vi "AOD Control (host).vi"() -> ()   [LabVIEW 2012]
uses:
  <vilib>/rvi/interface/nirviOpenFPGA/nirviOpenFPGA.xnode
  <vilib>/rvi/interface/nirviReadWriteControl/nirviReadWriteControl.xnode
  <vilib>/rvi/interface/nirviMethod/nirviMethod.xnode
  <vilib>/LabVIEW Targets/FPGA/RIO/nirio_PxiTriggers.ctl
  <vilib>/rvi/interface/nirviCloseFPGA/nirviCloseFPGA.xnode
  <resource>/objmgr/daqmx.rc
  <vilib>/Utility/error.llb/DialogType.ctl
  <vilib>/DAQmx/write.llb/DAQmx Write (Digital Bool 1Line 1Point).vi
  <instrlib>/niHWS/nihws.llb/niHWS Write Analog I32.vi
  <instrlib>/niHWS/nihws.llb/niHWS Open File Permissions ID.ctl
  <vilib>/DAQmx/create/channels.llb/DAQmx Create Channel (DO-Digital Output).vi
  <vilib>/DAQmx/read.llb/DAQmx Read (Raw 1D I32).vi
  <instrlib>/niHWS/nihws.llb/niHWS Write Analog I16.vi
  <vilib>/DAQmx/write.llb/DAQmx Write (Analog DBL 1Chan 1Samp).vi
  FPGA Bitfiles/AOD Control.lvproj_PXI-7954R_AOD Control (FPGA)~D2.lvbitx
  AOD Control (FPGA).vi
  AODRef.ctl
  <vilib>/Analysis/NI_AALBase.lvlib
  <vilib>/Analysis/1siggen.llb/Ramp Pattern by Samples.vi
  <vilib>/rvi/errors/niLvFpgaMergeErrorWithErrorCode.vi
  <vilib>/FPGA/interface/niFpgaViExecutionMode.ctl
  <vilib>/userdefined/High Color/nirio_resource_hc.ctl
panel:
  in  "Max":u32=700000
  in  "GridPoints":dbl=5.0
  in  "Power":dbl(slide) min=0.0 max=5.0 step=0.1 scale=0.0..5.0
  out "OutOfRange":bool
  out "Processing":bool
  out "Acquire":bool
  out "FPGA State":T1(ring)
  out "Host State":T2(ring)
  out "Scanning Your Mom":dbl(slide) scale=0.0..1.0
  in  "Tab Control":T3(tab)=enum."Miscellaneous"
  in  "Display Data":bool=TRUE
  in  "ClearPoints":bool
  in  "Scan Settings":T4={"XStart"=-200000000, "XEnd"=200000000, "XNum"=500, "YStart"=-200000000, "YEnd"=200000000, "YNum"=500, "ZStart"=0, "ZEnd"=0, "ZNum"=1}
  in  "Points":i32[][](array[numeric])
  in  "Stop":bool
  in  "Scan":bool
  in  "Volume Scan":bool
  in  "Abort":bool
  in  "Reset":bool
  out "Writing":bool
  in  "SaveStream":bool
  in  "SaveImage":bool
  in  "Path":path
  in  "Scans":i32=5
  in  "ImCh1":bool=TRUE
  in  "Ephys":bool
  in  "Photodiode":bool
  in  "ImCh2":bool
  in  "Throwaway (us)":i32=10
  out "PointArray":cluster{"X":i32, "Y":i32, "Z":i32}[](array[cluster])
  out "StreamInfo":T5
  in  "Downsample":i32=40
  in  "DDS SysClk":i32=100000000
  in  "FPGA Clk":i32=40000000
  in  "ImReadSize":i32=10000
  in  "AcqDivider":i32=20
  out "Acq Freq":dbl format="%#_8g"
  out "Loop Count":i32
  out "PointTime":u32
  out "PMT FIFO Space":u32
  out "ImCh Backlog":u32
  out "FPGA PMT Remaining":u32
  out "PMT Backlog":u32
  out "Command":i16
  in  "P high":u32=10
  in  "P":bool
  out "PMT Read":i32
  out "FPGA Loop Count":i32
  out "Point":cluster{"X":i32, "Y":i32, "Z":i32}
  out "TotalSamples":u32
  out "Written":cluster{"Address":u8, "Value":u32}[](array[cluster]) {"Address" format="%x"; "Value" format="%x"}
  out "PMT Array":i32[](array[numeric])
  out "ImCh Read":i32
  out "Mode":enum16{"Points", "Volume", "Idle"}(ring)
  out "FPGA VI Execution Mode":T6
  out "StackSize":cluster{"nX":u32, "nY":u32, "nZ":u32}
  out "raw out":refnum<queue>
  out "voxel queue":refnum<queue>
  out "NumChans":u32
  out "XPos":i32[](array[numeric])
  out "TRIG0":bool
  out "ExtAcqTrig":bool
  out "TriggerAcq":bool=TRUE
  out "Armed":bool
  out "Bad PMTData":bool
  out "SerialError":bool
  out "Sequencing error":bool
  out "YPos":i32[](array[numeric])
  out "ZPos":i32[](array[numeric])
  out "Point Freq":dbl
  out "SampleCount":u32
  out "AcqDivCount":u32
  out "# pending remove":i32
  out "Processed":i32
  in  "BlankTime (us)":i16=10
  out "BlankSamples":u32
  out "Throwaway Samples":dbl
  out "RepNum":i32
  out "NumReps":i32
  out "NumPoints":i32
  out "PointNum":u32
  out "LaserPowerTask":refnum<k21>
  in  "Execute":bool
  in  "Debug Mode":T7(ring)
  in  "Space":i32
  in  "decimating factor":i32=10
  in  "BaselineRate":dbl=0.01 min=0.0 max=1.0
  in  "RIO Device":T8="RIO0"
  out "ImData":i32[][](array[numeric])
  out "ImCh1 2":T9(plugin-control)
  out "ImCh2 2":T9(plugin-control)
  in  "Section":i32(c297)
  out "Waveform Chart":waveform(dbl)[](graph)
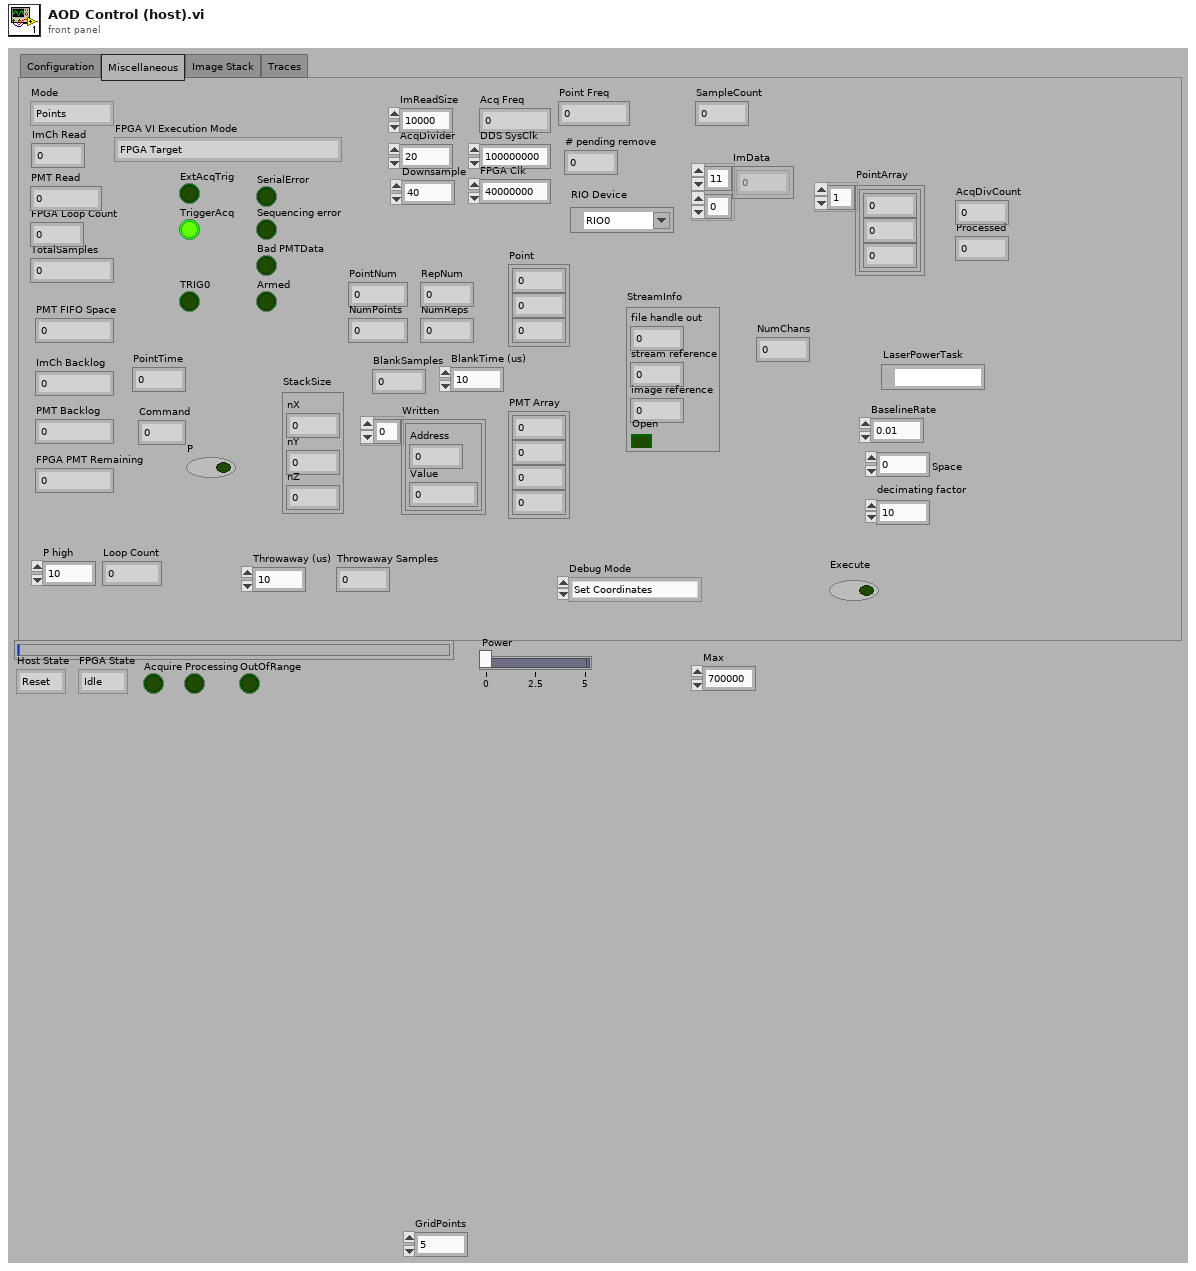
[diagram p1: front panel]
types:
  T1 = enum16{"Idle", "Write Registers", "Receive Points", "Prepare Volume", "Arm Scan", "Scan Points"}
  T2 = enum16{"Reset", "Idle", "Start Acquire", "Acquire", "End Acquire"}
  T3 = enum32{"Configuration", "Miscellaneous", "Image Stack", "Traces"}
  T4 = cluster{"XStart":i32, "XEnd":i32, "XNum":i32, "YStart":i32, "YEnd":i32, "YNum":i32, "ZStart":i32, "ZEnd":i32, "ZNum":i32}
  T5 = cluster{"file handle out":u32, "stream reference":u32, "image reference":u32, "Open":bool}
  T6 = typedef "niFpgaViExecutionMode.ctl" = enum16{"FPGA Target", "Development Computer with Simulated I/O", "Development Computer with Real I/O", "Third-Party Simulator"}
  T7 = enum16{"Set Coordinates", "Toggle Axis", "Sweep Settings"}
  T8 = typedef "nirio_resource_hc.ctl" = tag
  T9 = typedef "IMAQ Image.ctl" = refnum<image>
  T10 = typedef "AODRef.ctl" = refnum<k20>
  T11 = typedef "nirio_PxiTriggers.ctl" = u16
  T12 = typedef "niHWS Open File Permissions ID.ctl" = enum32{"Read Only", "Read/Write Existing", "Read/Write/Create New", "Read/Write/Create New Always"}
  T13 = typedef "Image Type" = u32
  T14 = typedef "DialogType.ctl" = u16
  T15 = cluster{"Global Rectangle":i32[], "Contours":cluster{"Contour Type":u32, "ROI Type":u32, "Points":i32[]}[]}
  T16 = cluster{"Global Rectangle":i32[], "Contours":cluster{"Contour Type":u32, "ROI Type":u32, "Points":i32[]}[]}[]
  T17 = cluster{"Contour Type":u32, "ROI Type":u32, "Points":i32[]}[]
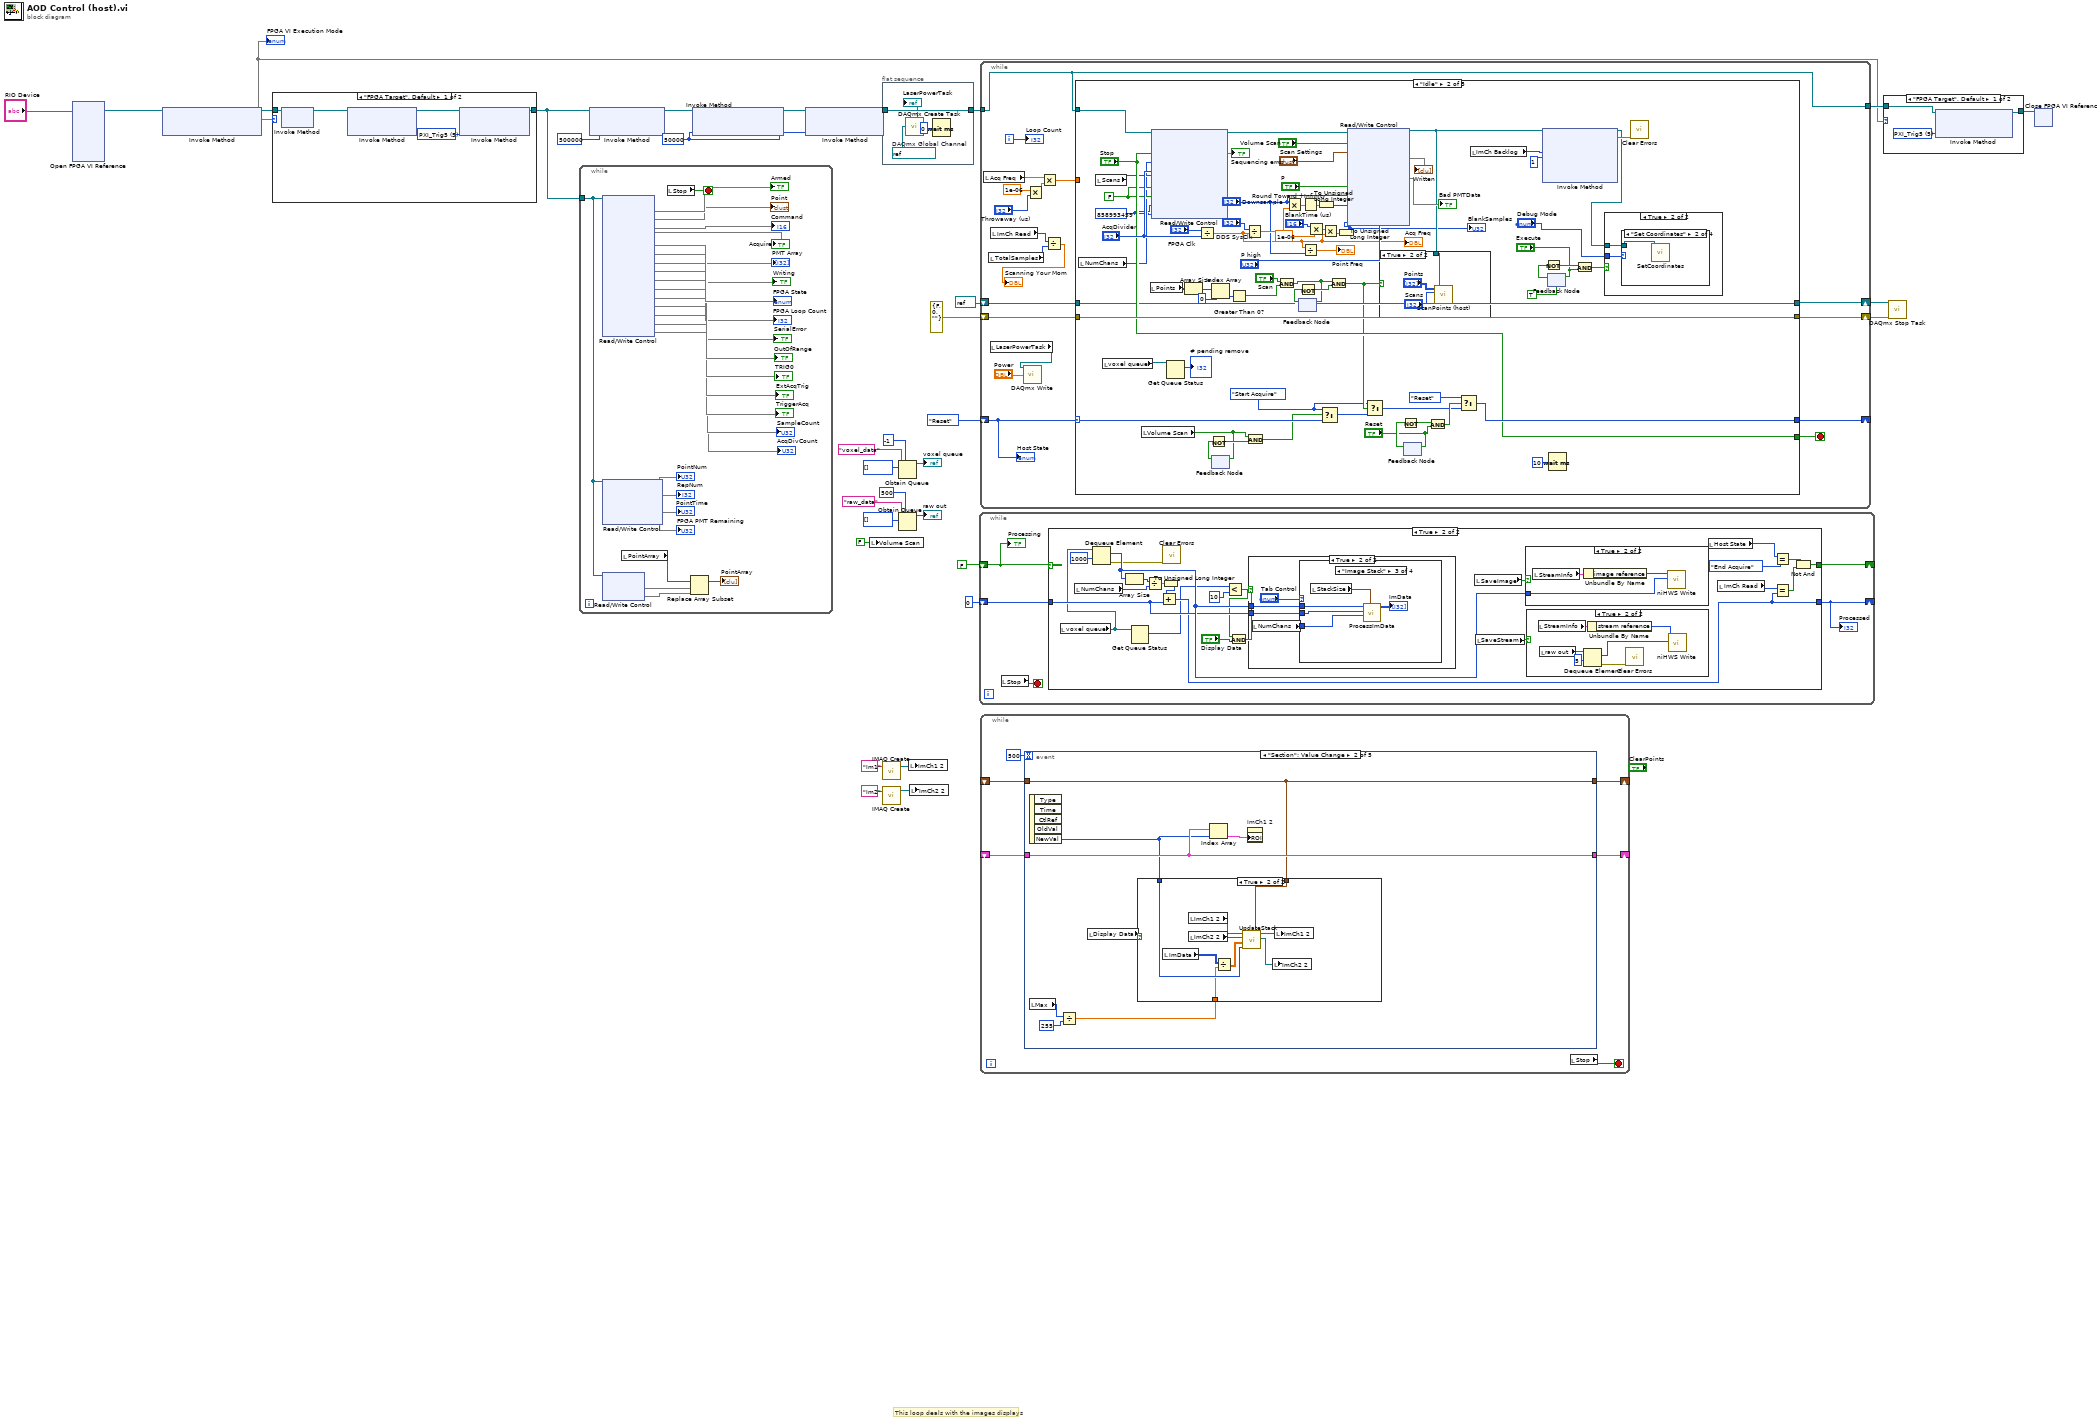
[diagram p0: block diagram]
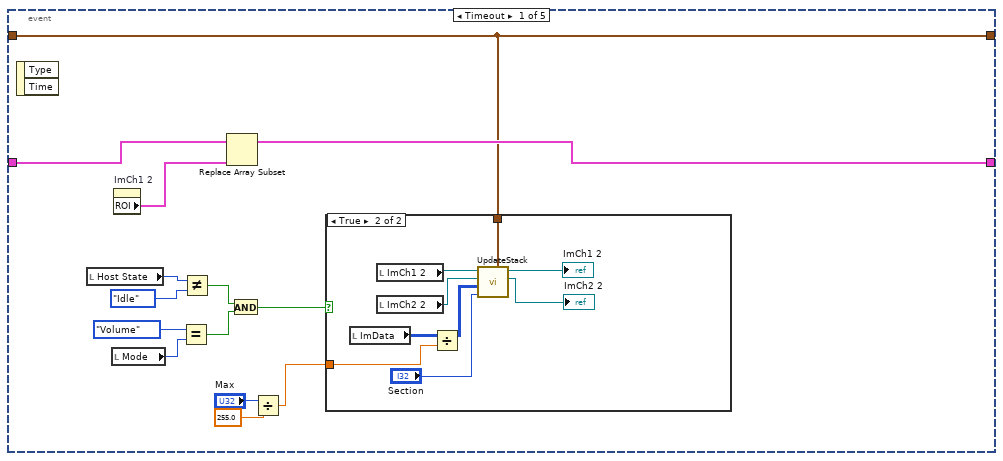
[diagram p2: hidden frame]
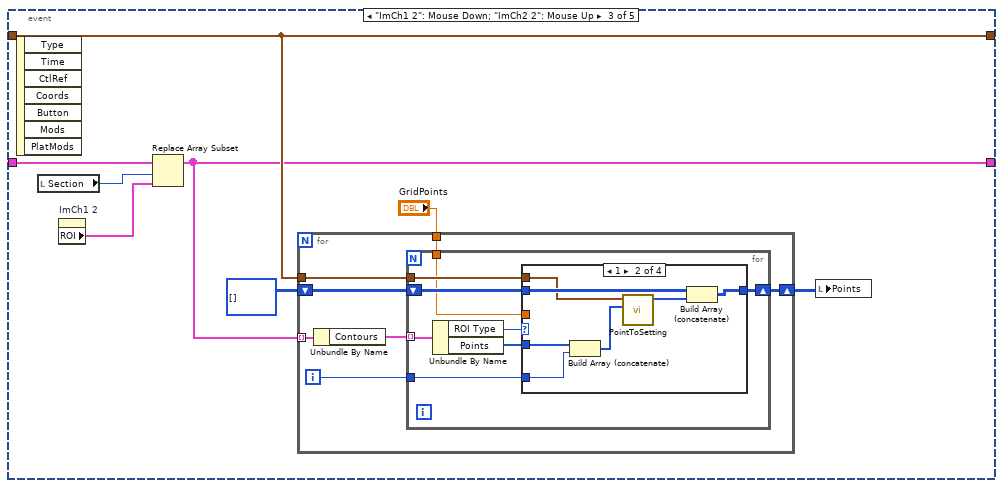
[diagram p5: hidden frame]
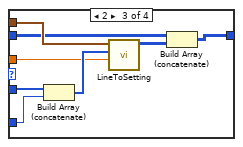
[diagram p7: hidden frame]
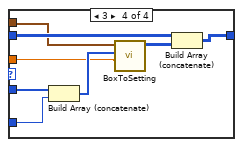
[diagram p8: hidden frame]
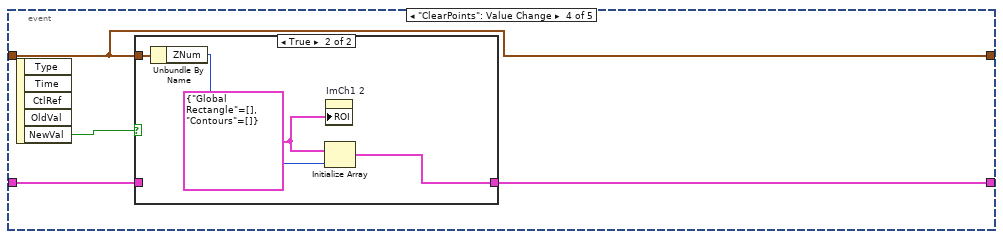
[diagram p9: hidden frame]
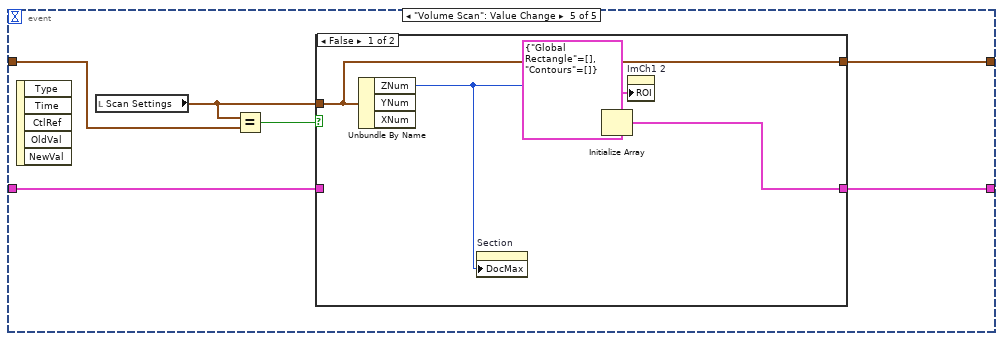
[diagram p11: hidden frame]
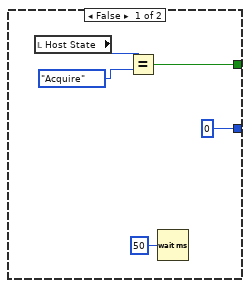
[diagram p13: hidden frame]
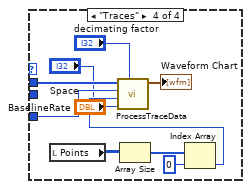
[diagram p19: hidden frame]
diagram:
  w29 = u32 50000 ("Depth")
  # "This loop deals with the images displays"
  n1 = xnode "Open FPGA VI Reference"("resource name"="RIO Device") -> ("FPGA VI Reference Out"=w33:T10)  [unwired: 1 in, 1 out]
  n2 = xnode "Invoke Method"("FPGA VI Reference In"=w33) -> ("FPGA VI Reference Out"=w20:T10, "FPGA VI Execution Mode"=w19)  [unwired: 1 in, 1 out]
  "FPGA VI Execution Mode" <- w19
  n3 = case shown="\"FPGA Target\", Default" w19 {
    tunnel: [w34 w39] -> w7
    tunnel: w20 -> [w38 w39]
    frame "FPGA Target", Default {
      w36 = T11 5 items=["PXI_Trig0", "PXI_Trig1", "PXI_Trig2", "PXI_Trig3", "PXI_Trig4", "PXI_Trig5", "PXI_Trig6", "PXI_Trig7"] ("Trigger")
      n4 = xnode "Invoke Method"("FPGA VI Reference In"=w38) -> ("FPGA VI Reference Out"=w37:T10)  [unwired: 1 in, 1 out]
      n5 = xnode "Invoke Method"("FPGA VI Reference In"=w37) -> ("FPGA VI Reference Out"=w35:T10)  [unwired: 2 in, 1 out]
      n6 = xnode "Invoke Method"("FPGA VI Reference In"=w35, "Trigger"=w36) -> ("FPGA VI Reference Out"=w34:T10)  [unwired: 1 in, 1 out]
    }
    frame "Development Computer with Simulated I/O" {
    }
  }
  n7 = while {
    tunnel: w7 -> [w46]
    stop <- w64 stop-if-true
    n8 = xnode "Read/Write Control"("FPGA VI Reference In"=w46) -> ("Armed"=→"Armed", "Point"=→"Point", "Command"=→"Command", "Acquire"=→"Acquire", "PMT Array"=→"PMT Array", "Writing"=→"Writing", "State"=→"FPGA State", "Count"=→"FPGA Loop Count", "SerialError"=→"SerialError", "OutOfRange"=→"OutOfRange", "TRIG0"=→"TRIG0", "ExtAcqTrig"=→"ExtAcqTrig", "TriggerAcq"=→"TriggerAcq", "SampleCount"=→"SampleCount", "AcqDivCount"=→"AcqDivCount")  [unwired: 1 in, 2 out]
    n9 = xnode "Read/Write Control"("FPGA VI Reference In"=w46) -> ("PointNum"=→"PointNum", "RepNum"=→"RepNum", "PointTime"=→"PointTime", "PMT Remaining"=→"FPGA PMT Remaining")  [unwired: 1 in, 2 out]
    n10 = xnode "Read/Write Control"("FPGA VI Reference In"=w46) -> ("PointNum"=w43, "Point"=w42)  [unwired: 1 in, 2 out]
    n11 = local read "PointArray"() -> (w45:cluster{"X":i32, "Y":i32, "Z":i32}[])
    n12 = local read "Stop"() -> (w64:bool)
    n13 = Replace Array Subset(array=w45, new element=w42, index=w43) -> (→"PointArray":cluster{"X":i32, "Y":i32, "Z":i32}[])
  }
  n14 = xnode "Invoke Method"("FPGA VI Reference In"=w7, "Depth"=u32 500000) -> ("FPGA VI Reference Out"=w22:T10)  [unwired: 1 in, 1 out]
  n15 = xnode "Invoke Method"("FPGA VI Reference In"=w22, "Depth"=w29) -> ("FPGA VI Reference Out"=w21:T10)  [unwired: 1 in, 1 out]
  n16 = xnode "Invoke Method"("FPGA VI Reference In"=w21, "Depth"=w29) -> ("FPGA VI Reference Out"=w24:T10)  [unwired: 1 in, 1 out]
  n17 = local write "Volume Scan"(FALSE ("Volume Scan")) -> ()
  n18 = call "IMAQ Create"("Image Name"="Im1") -> ("New Image"=w2:T9)  [unwired: 4 in, 1 out]
  n19 = call "IMAQ Create"("Image Name"="Im2") -> ("New Image"=w1:T9)  [unwired: 4 in, 1 out]
  n20 = flat-sequence {
    tunnel: [w68] -> w23
    tunnel: w24 -> [w68]
    frame #0 {
      w65 = refnum<k21> "AOD Gain"  # DAQmx Global Channel
      n21 = call <vilib>:"DAQmx Create Task.vi"("global virtual channels"=w65) -> ("task out"=→"LaserPowerTask":refnum<k21>)  [unwired: 4 in, 10 out]
      n22 = Wait (ms)(milliseconds to wait=u32 0) -> ()  [unwired: 1 out]
    }
  }
  n23 = Obtain Queue(max queue size (-1, unlimited)=-1, name (unnamed)="voxel_data", element data type=u32[] [] ("data")) -> (queue out=→"voxel queue":refnum<queue>)  [unwired: 2 in, 2 out]
  n24 = Obtain Queue(max queue size (-1, unlimited)=500, name (unnamed)="raw_data", element data type=u32[] [] ("data")) -> (queue out=→"raw out":refnum<queue>)  [unwired: 2 in, 2 out]
  n25 = local write "ImCh1 2"(w2) -> ()
  n26 = local write "ImCh2 2"(w1) -> ()
  n27 = while {
    shift-right: [w69] -> _
    shift-left: 0 -> [w72]
    shift-right: [w71] -> _
    shift-left: FALSE -> [w70]
    stop <- w73 stop-if-true
    n28 = local read "Stop"() -> (w73:bool)
    n29 = case shown="True" w70 {
      tunnel: w72 -> [_ w95]
      tunnel: [0 w91] -> w69
      tunnel: [w74 w90] -> w71
      frame False {
        n30 = local read "Host State"() -> (w75:T2)
        n31 = Equal?(x=w75, y=T2."Acquire") -> (x = y?=w74:bool)
        n32 = Wait (ms)(milliseconds to wait=u32 50) -> ()  [unwired: 1 out]
      }
      frame True {
        n33 = local read "voxel queue"() -> (w86:refnum<queue>)
        n34 = local read "NumChans"() -> (w84:u32)
        n35 = Dequeue Element(queue=w86, timeout in ms (-1)=1000) -> (element=w99:u32[], error out=w96:errorcluster)  [unwired: 1 in, 2 out]
        n36 = Array Size(array=w99) -> (size(s)=w85:i32)
        n37 = Get Queue Status(queue=w86) -> (# pending remove=w87:i32)  [unwired: 2 in, 7 out]
        n38 = Divide(x=w85, y=w84) -> (x/y=w83:dbl)
        n39 = To Unsigned Long Integer(number=w83) -> (unsigned 32bit integer=w82:u32)
        n40 = Add(x=w82, y=w95) -> (x+y=w91:u32)
        n41 = call <vilib>:"Clear Errors.vi"("error in (no error)"=w96) -> ()  [unwired: 6 in, 1 out]
        n42 = Less?(x=w87, y=10) -> (x < y?=w80:bool)
        n43 = And(x=w80, y="Display Data") -> (x .and. y?=w79:bool)
        n44 = case shown="True" w79 {
          tunnel: w99 -> [_ w113]
          tunnel: w95 -> [_ w112]
          frame False {
          }
          frame True {
            n45 = local read "NumChans"() -> (w111:u32)
            n46 = case shown="\"Image Stack\"" "Tab Control" {
              tunnel: w113 -> [_ _ w119 w129]
              tunnel: w112 -> [_ _ w118 _]
              tunnel: w111 -> [_ _ w116 w128]
              frame "Configuration", Default {
              }
              frame "Miscellaneous" {
              }
              frame "Image Stack" {
                n47 = local read "StackSize"() -> (w117:cluster{"nX":u32, "nY":u32, "nZ":u32})
                n48 = call "ProcessImData.vi"("StackSize"=w117, "NumChans"=w116, "StartingNum"=w118, "Data"=w119) -> ("output array"=→"ImData":i32[][])  [unwired: 7 in]
              }
              frame "Traces" {
                n49 = local read "Points"() -> (w127:i32[][])
                n50 = Array Size(array=w127) -> (size(s)=w126:i32[])
                n51 = Index Array(array=w126, index=0) -> (element=w124:i32)
                n52 = call "ProcessTraceData.vi"("BaselineRate"="BaselineRate", "decimating factor"="decimating factor", "Space"="Space", "NumPoints"=w124, "NumChans"=w128, "Data"=w129) -> ("Waveforms"=→"Waveform Chart":waveform(dbl)[])  [unwired: 5 in]
              }
            }
          }
        }
        n53 = local read "SaveImage"() -> (w100:bool)
        n54 = local read "SaveStream"() -> (w98:bool)
        n55 = case shown="True" w100 {
          tunnel: w99 -> [_ w108]
          frame False {
          }
          frame True {
            n56 = local read "StreamInfo"() -> (w110:T5)
            n57 = Unbundle By Name(w110) -> ("image reference"=w109:u32)
            n58 = call-poly <instrlib>:"niHWS Write.vi"("data"=w108, "waveform reference in"=w109) -> ()  [unwired: 8 in, 2 out]
          }
        }
        n59 = case shown="True" w98 {
          frame False {
          }
          frame True {
            n60 = local read "StreamInfo"() -> (w107:T5)
            n61 = local read "raw out"() -> (w105:refnum<queue>)
            n62 = Dequeue Element(queue=w105, timeout in ms (-1)=5) -> (element=w104:u32[], error out=w102:errorcluster)  [unwired: 1 in, 2 out]
            n63 = Unbundle By Name(w107) -> ("stream reference"=w106:u32)
            n64 = call <vilib>:"Clear Errors.vi"("error in (no error)"=w102) -> ()  [unwired: 6 in, 1 out]
            n65 = call-poly <instrlib>:"niHWS Write.vi"("data"=w104, "waveform reference in"=w106) -> ()  [unwired: 8 in, 2 out]
          }
        }
        n66 = local read "Host State"() -> (w93:T2)
        n67 = local read "ImCh Read"() -> (w92:i32)
        n68 = Equal?(x=w93, y=T2."End Acquire") -> (x = y?=w89:bool)
        n69 = Equal?(x=w92, y=w91) -> (x = y?=w88:bool)
        n70 = Not And(1:w88, 2:w89) -> (0:w90:bool)
      }
    }
    "Processed" <- w69
    "Processing" <- w70
  }
  n71 = while {
    tunnel: w23 -> [w140]
    tunnel: [w140] -> w30
    shift-right: [w142] -> _
    shift-left: T2."Reset" -> [w143]
    shift-right: [w147] -> w28
    shift-left: refnum<k21> refnum ("task out") -> [w145]
    shift-right: [w146] -> w27
    shift-left: errorcluster {"status"=FALSE, "code"=0, "source"=""} ("error out") -> [w144]
    i -> [w148]
    stop <- w141 stop-if-true
    n72 = local read "Acq Freq"() -> (w133:dbl)
    n73 = local read "TotalSamples"() -> (w138:u32)
    n74 = local read "LaserPowerTask"() -> (w131:refnum<k21>)
    n75 = local read "ImCh Read"() -> (w139:i32)
    n76 = call-poly <vilib>:"DAQmx Write.vi"("task/channels in"=w131, "data"="Power") -> ()  [unwired: 11 in, 3 out]
    n77 = Multiply(x=1e-06, y="Throwaway (us)") -> (x*y=w134:dbl)
    n78 = Multiply(x=w133, y=w134) -> (x*y=w132:dbl)
    n79 = Divide(x=w139, y=w138) -> (x/y=→"Scanning Your Mom":dbl)
    n80 = case shown="\"Idle\"" w143 {
      selector: w143 -> [_ w287 _ _ _]
      tunnel: w144 -> [w172 w286 w298 w544 w656]
      tunnel: w145 -> [w171 w261 w299 w545 w650]
      tunnel: [w168 w261 w296 w558 w650] -> w147
      tunnel: [w169 w286 w297 w546 w651] -> w146
      tunnel: [T2."Idle" w275 T2."Acquire" w557 w649] -> w142
      tunnel: w140 -> [w165 w276 w300 w530 w653]
      tunnel: [FALSE ("Stop") "Stop" FALSE ("Stop") FALSE ("Stop") FALSE ("Stop")] -> w141
      tunnel: w132 -> [_ _ _ w519 _]
      frame "Reset" {
        w149 = tag ""  # DAQmx Physical Channel
        w150 = tag "PXI1Slot2/ai3"  # DAQmx Physical Channel
        w151 = tag "PXI1Slot2/ai2"  # DAQmx Physical Channel
        w152 = tag "PXI1Slot2/ai1"  # DAQmx Physical Channel
        w153 = tag "PXI1Slot2/ai0"  # DAQmx Physical Channel
        w170 = cluster{"Address":u8, "Value":u32}[] [{"Address"=0, "Value"=240}, {"Address"=1, "Value"=13762560}, {"Address"=2, "Value"=0}, {"Address"=3, "Value"=8413952}, {"Address"=4, "Value"=0}, {"Address"=5, "Value"=0}, {"Address"=6, "Value"=1023}, {"Address"=7, "Value"=257}, {"Address"=8, "Value"=0}, {"Address"=9, "Value"=0}, {"Address"=0, "Value"=246}]  # Initialization Vector
        (unwired) cluster{"Address":u8, "Value":u32}[] [{"Address"=0, "Value"=240}, {"Address"=1, "Value"=13762592}, {"Address"=2, "Value"=32768}, {"Address"=3, "Value"=8413952}, {"Address"=4, "Value"=0}, {"Address"=5, "Value"=0}, {"Address"=6, "Value"=1023}, {"Address"=7, "Value"=257}, {"Address"=8, "Value"=21}, {"Address"=4, "Value"=858993459}]  # Initialization Vector
        # "This is necessary in the case of an abort, where \nthe acquire loop stops before all the image data\nhas been pulled from the FIFO"
        n81 = stacked-sequence {
          tunnel: w165 -> [_ w196 w202 w210 w215]
          tunnel: w170 -> [_ _ w199 _ _]
          frame #0 {
            n82 = local write "Acquire"(FALSE ("Acquire")) -> ()
            n83 = Wait (ms)(milliseconds to wait=u32 50) -> ()  [unwired: 1 out]
          }
          frame #1 {
            n84 = xnode "Read/Write Control"("FPGA VI Reference In"=w196, "Abort"=FALSE, "Reset"=TRUE) -> ()  [unwired: 1 in, 2 out]
            n85 = Wait (ms)(milliseconds to wait=u32 10) -> ()  [unwired: 1 out]
          }
          frame #2 {
            n86 = Wait (ms)(milliseconds to wait=u32 500) -> ()  [unwired: 1 out]
            n87 = Array Size(array=w199) -> (size(s)=w205:i32)
            n88 = xnode "Read/Write Control"("FPGA VI Reference In"=w202, "Register Writes"=w199, "Number Registers"=w205, "Write Register"=FALSE, "WriteSize"=enum16{"1", "2", "4"}."1", "SclkDivider"=u32 4 ("ClockPause"), "stop"=FALSE, "Downsample"=40, "Reset"=FALSE, "PMT Timeout"=20000000) -> ()  [unwired: 1 in, 2 out]
          }
          frame #3 {
            n89 = xnode "Read/Write Control"("FPGA VI Reference In"=w210, "Write Register"=TRUE) -> ()  [unwired: 1 in, 2 out]
            n90 = Wait (ms)(milliseconds to wait=u32 10) -> ()  [unwired: 1 out]
          }
          frame #4 {
            n91 = xnode "Read/Write Control"("FPGA VI Reference In"=w215, "Write Register"=FALSE, "WriteSize"=enum16{"1", "2", "4"}."4", "SclkDivider"=u32 2 ("ClockPause"), "Pause"=u32 4, "UpdateIO time"=u32 4) -> ()  [unwired: 1 in, 2 out]
          }
        }
        n92 = Select(t=w153, s="ImCh1", f=w149) -> (s? t:f=w156:tag)
        n93 = Select(t=w152, s="ImCh2", f=w149) -> (s? t:f=w155:tag)
        n94 = Select(t=w151, s="Photodiode", f=w149) -> (s? t:f=w159:tag)
        n95 = Select(t=w150, s="Ephys", f=w149) -> (s? t:f=w161:tag)
        n96 = Build Array(w156, w155, w159, w161) -> (w163:tag[])
        n97 = call <vilib>:"DAQmx Flatten Channel String.vi"("names in"=w163) -> ("names out"=w154:string)  [unwired: 13 in, 1 out]
        n98 = local read "FPGA VI Execution Mode"() -> (w167:T6)
        n99 = case shown="\"FPGA Target\", Default" w167 {
          tunnel: w172 -> [w189 w191]
          tunnel: w171 -> [w188 w192]
          tunnel: [w183 w191] -> w169
          tunnel: [w184 w192] -> w168
          tunnel: [w182 u32 1 ("NumChans")] -> w166
          tunnel: w154 -> [w181 _]
          frame "FPGA Target", Default {
            n100 = call <vilib>:"DAQmx Clear Task.vi"("task in"=w188, "error in"=w189) -> ("error out"=w187:errorcluster)  [unwired: 13 in]
            n101 = call <vilib>:"Clear Errors.vi"("error in (no error)"=w187) -> ()  [unwired: 6 in, 1 out]
            n102 = call "ConfigureAcqTask.vi"("AcqCh"=w181) -> ("error out"=w185:errorcluster, "task out"=w186:refnum<k21>)  [unwired: 9 in]
            n103 = property class="DAQmx Read"(reference=w186, error in=w185) -> (reference out=w184:refnum<k21>, error out=w183:errorcluster, "NumChans"=w182:u32)
          }
          frame "Development Computer with Simulated I/O" {
          }
        }
        "NumChans" <- w166
        n104 = while {
          tunnel: w165 -> [w180]
          shift-right: [w175] -> _
          shift-left: u32 1 ("Number of Elements") -> [w176]
          stop <- w179 stop-if-true
          n105 = xnode "Invoke Method"("FPGA VI Reference In"=w180, "Number of Elements"=w176, "Timeout (ms)"=5) -> ("error out"=w177:errorcluster, "Elements Remaining"=w175)  [unwired: 1 in, 2 out]
          n106 = Equal To 0?(x=w175) -> (x = 0?=w179:bool)
          n107 = call <vilib>:"Clear Errors.vi"("error in (no error)"=w177) -> ()  [unwired: 6 in, 1 out]
        }
      }
      frame "Idle" {
        w219 = u32 858993459 ("LP Center Frequency")
        w252 = FALSE
        w248 = T2."Start Acquire"
        n108 = local read "NumChans"() -> (w246:u32)
        n109 = local read "Scans"() -> (w253:i32)
        n110 = local read "voxel queue"() -> (w242:refnum<queue>)
        n111 = local read "Volume Scan"() -> (w255:bool)
        n112 = local read "Points"() -> (w239:i32[][])
        n113 = xnode "Read/Write Control"("FPGA VI Reference In"=w276, "stop"="Stop", "Channels"=w246, "AcqDivider"="AcqDivider", "NumReps"=w253, "TriggerAcq"=w252, "ExtAcqTrig"=w252, "HP Center Frequency"=w219, "LP Center Frequency"=w219) -> ("FPGA VI Reference Out"=w281:T10, "Sequencing error"=→"Sequencing error")  [unwired: 1 in, 1 out]
        n114 = Get Queue Status(queue=w242) -> (# pending remove=→"# pending remove":i32)  [unwired: 2 in, 7 out]
        n115 = Array Size(array=w239) -> (size(s)=w238:i32[])
        n116 = Divide(x="FPGA Clk", y="AcqDivider") -> (x/y=w232:dbl)
        "Acq Freq" <- w232
        n117 = Index Array(array=w238, index=0) -> (element=w236:i32)
        n118 = feedback-in #1(w255) -> ()
        n119 = feedback #1() -> (w257:bool)  [unwired: 1 in]
        n120 = Not(x=w257) -> (.not. x?=w256:bool)
        n121 = Greater Than 0?(x=w236) -> (x > 0?=w234:bool)
        n122 = Divide(x="DDS SysClk", y=w232) -> (x/y=w268:dbl)
        n123 = And(x=w255, y=w256) -> (x .and. y?=w254:bool)
        n124 = And(x="Scan", y=w234) -> (x .and. y?=w233:bool)
        n125 = Multiply(x="Downsample", y=w268) -> (x*y=w270:dbl)
        n126 = feedback-in #2(w233) -> ()
        n127 = feedback #2() -> (w265:bool)  [unwired: 1 in]
        n128 = Not(x=w265) -> (.not. x?=w266:bool)
        n129 = Round Toward +Infinity(x=w270) -> (ceil(x): smallest int >= x=w269:dbl)
        n130 = Divide(x=w232, y="Downsample") -> (x/y=→"Point Freq":dbl)
        n131 = Multiply(x="BlankTime (us)", y=1e-06) -> (x*y=w231:dbl)
        n132 = To Unsigned Long Integer(number=w269) -> (unsigned 32bit integer=w262:u32)
        n133 = Select(t=w248, s=w254, f=w287) -> (s? t:f=w249:T2)
        n134 = Multiply(x=w231, y=w232) -> (x*y=w228:dbl)
        n135 = And(x=w233, y=w266) -> (x .and. y?=w250:bool)
        n136 = To Unsigned Long Integer(number=w228) -> (unsigned 32bit integer=w227:u32)
        "BlankSamples" <- w227
        n137 = xnode "Read/Write Control"("FPGA VI Reference In"=w281, "Volume Scan"="Volume Scan", "Scan Settings"="Scan Settings", "P"="P", "Downsample"="Downsample", "UpdatesPerPoint"=w262, "P high"="P high", "BlankSamples"=w227) -> ("FPGA VI Reference Out"=w245:T10, "Written"=→"Written", "Bad PMTData"=→"Bad PMTData")  [unwired: 1 in, 2 out]
        n138 = Select(t=w248, s=w250, f=w249) -> (s? t:f=w247:T2)
        n139 = case shown="True" w250 {
          tunnel: w245 -> [_ w293]
          frame False {
          }
          frame True {
            n140 = call "ScanPoints (host).vi"(7:w293, "Points"="Scans", "FPGA VI Reference Out"="Points") -> ()  [unwired: 9 in]
          }
        }
        n141 = feedback-in #3("Reset") -> ()
        n142 = feedback #3() -> (w273:bool)  [unwired: 1 in]
        n143 = Not(x=w273) -> (.not. x?=w272:bool)
        n144 = And(x=w272, y="Reset") -> (x .and. y?=w271:bool)
        n145 = Select(t=T2."Reset", s=w271, f=w247) -> (s? t:f=w275:T2)
        n146 = local read "ImCh Backlog"() -> (w263:u32)
        n147 = xnode "Invoke Method"("FPGA VI Reference In"=w245, "Number of Elements"=w263, "Timeout (ms)"=1) -> ("FPGA VI Reference Out"=w221:T10, "error out"=w264:errorcluster)  [unwired: 1 in, 2 out]
        n148 = feedback-in #4("Execute") -> ()
        n149 = feedback #4(TRUE ("Sweep")) -> (w225:bool)
        n150 = Not(x=w225) -> (.not. x?=w224:bool)
        n151 = Wait (ms)(milliseconds to wait=u32 10) -> ()  [unwired: 1 out]
        n152 = And(x=w224, y="Execute") -> (x .and. y?=w222:bool)
        n153 = case shown="True" w222 {
          tunnel: w221 -> [_ w288]
          tunnel: "Debug Mode" -> [_ w289]
          frame False {
          }
          frame True {
            n154 = case shown="\"Set Coordinates\"" w289 {
              tunnel: w288 -> [_ w290 w291 w292]
              frame Default {
              }
              frame "Set Coordinates" {
                n155 = call "SetCoordinates.vi"("FPGA VI Reference Out"=w290) -> ()  [unwired: 11 in]
              }
              frame "Sweep Settings" {
                n156 = call "SweepSettings.vi"("FPGA VI Reference Out"=w291) -> ()  [unwired: 11 in]
              }
              frame "Toggle Axis" {
                n157 = call "ToggleAxis.vi"("FPGA VI Reference Out"=w292) -> ()  [unwired: 11 in]
              }
            }
          }
        }
        n158 = call <vilib>:"Clear Errors.vi"("error in (no error)"=w264) -> ()  [unwired: 6 in, 1 out]
      }
      frame "Start Acquire" {
        n159 = stacked-sequence {
          tunnel: w300 -> [w307 _ w434]
          tunnel: w299 -> [_ _ w433]
          tunnel: w298 -> [_ _ w432]
          tunnel: [_ _ w431] -> w297
          tunnel: [_ _ w430] -> w296
          frame #0 {
            w308 = 0 ("PMT Read")
            w304 = FALSE ("Volume Scan")
            n160 = local read "voxel queue"() -> (w306:refnum<queue>)
            n161 = local read "raw out"() -> (w305:refnum<queue>)
            n162 = xnode "Read/Write Control"("FPGA VI Reference In"=w307) -> ("FPGA VI Reference Out"=w312:T10, "NumPoints"=→"NumPoints", "NumReps"=→"NumReps", "Mode"=w313)  [unwired: 1 in, 1 out]
            "Mode" <- w313
            n163 = local write "Volume Scan"(w304) -> ()
            n164 = local write "Scan"(w304) -> ()
            n165 = local write "PMT Read"(w308) -> ()
            n166 = local write "ImCh Read"(w308) -> ()
            n167 = Flush Queue(queue=w306) -> ()  [unwired: 1 in, 3 out]
            n168 = Flush Queue(queue=w305) -> ()  [unwired: 1 in, 3 out]
            n169 = case shown="\"Volume\"" w313 {
              tunnel: w312 -> [_ w331]
              tunnel: [w322 w330] -> w315
              tunnel: [w318 w328] -> w316
              tunnel: [w320 w326] -> w309
              tunnel: [w318 w329] -> w303
              frame "Points", Default {
                w318 = 0
                n170 = local read "Points"() -> (w325:i32[][])
                n171 = Array Size(array=w325) -> (size(s)=w324:i32[])
                n172 = local write "Tab Control"(T3."Traces" ("Tab Control")) -> ()
                n173 = Index Array(array=w324, index=0) -> (element=w322:i32)
                n174 = local read "Scans"() -> (w321:i32)
                n175 = Multiply(x=w322, y=w321) -> (x*y=w320:i32)
              }
              frame "Volume" {
                n176 = stacked-sequence {
                  tunnel: w331 -> [w335 w347 w364]
                  frame #0 {
                    n177 = xnode "Read/Write Control"("FPGA VI Reference In"=w335) -> ("Scan Settings.XEnd"=w340, "Scan Settings.XStart"=w336, "Scan Settings.XNum"=w338)  [unwired: 1 in, 2 out]
                    n178 = Subtract(x=w340, y=w336) -> (x-y=w339:dbl)
                    n179 = Quotient & Remainder(x=w339, y=w338) -> (floor(x/y)=w337:dbl)  [unwired: 1 out]
                    n180 = for {
                      N: w338 -> [_]
                      tunnel: w337 -> [w344]
                      tunnel: w336 -> [w342]
                      tunnel: [w341] -> w334 mode=indexing
                      i -> [w345]
                      n181 = Multiply(x=w344, y=w345) -> (x*y=w343:i32)
                      n182 = Add(x=w342, y=w343) -> (x+y=w341:i32)
                    }
                    "XPos" <- w334
                  }
                  frame #1 {
                    n183 = xnode "Read/Write Control"("FPGA VI Reference In"=w347) -> ("Scan Settings.YEnd"=w352, "Scan Settings.YStart"=w348, "Scan Settings.YNum"=w350)  [unwired: 1 in, 2 out]
                    n184 = Subtract(x=w352, y=w348) -> (x-y=w351:dbl)
                    n185 = Quotient & Remainder(x=w351, y=w350) -> (floor(x/y)=w349:dbl)  [unwired: 1 out]
                    n186 = for {
                      N: w350 -> [_]
                      tunnel: w349 -> [w356]
                      tunnel: w348 -> [w354]
                      tunnel: [w353] -> w346 mode=indexing
                      i -> [w357]
                      n187 = Multiply(x=w356, y=w357) -> (x*y=w355:i32)
                      n188 = Add(x=w354, y=w355) -> (x+y=w353:i32)
                    }
                    "YPos" <- w346
                  }
                  frame #2 {
                    n189 = xnode "Read/Write Control"("FPGA VI Reference In"=w364) -> ("Scan Settings.ZEnd"=w363, "Scan Settings.ZStart"=w359, "Scan Settings.ZNum"=w361)  [unwired: 1 in, 2 out]
                    n190 = Subtract(x=w363, y=w359) -> (x-y=w362:dbl)
                    n191 = Quotient & Remainder(x=w362, y=w361) -> (floor(x/y)=w360:dbl)  [unwired: 1 out]
                    n192 = for {
                      N: w361 -> [_]
                      tunnel: w360 -> [w368]
                      tunnel: w359 -> [w366]
                      tunnel: [w365] -> w358 mode=indexing
                      i -> [w369]
                      n193 = Multiply(x=w368, y=w369) -> (x*y=w367:i32)
                      n194 = Add(x=w366, y=w367) -> (x+y=w365:i32)
                    }
                    "ZPos" <- w358
                  }
                }
                n195 = local read "NumChans"() -> (w332:u32)
                n196 = xnode "Read/Write Control"("FPGA VI Reference In"=w331) -> ("Scan Settings.XNum"=w330, "Scan Settings.YNum"=w329, "Scan Settings.ZNum"=w328)  [unwired: 1 in, 2 out]
                n197 = for {
                  N: w328 -> [_]
                  tunnel: [w372] -> _ mode=indexing
                  tunnel: w332 -> [w370]
                  i -> [w371]
                  n198 = for {
                    N: w370 -> [_]
                    tunnel: [w378] -> w372 mode=indexing
                    tunnel: w371 -> [w377]
                    i -> [w376]
                    w373 = T13 0 items=["Grayscale (U8)", "Grayscale (I16)", "Grayscale (SGL)", "Complex (CSG)", "RGB (U32)", "HSL (U32)", "RGB (U64)", "Grayscale (U16)"] ("Image Type")
                    n199 = Format Into String(format string="%u_%u", w377, w376) -> (resulting string=w374:string)  [unwired: 2 in, 1 out]
                    n200 = call "IMAQ Create"("Image Name"=w374, "Image Type"=w373) -> ("New Image"=w378:T9)  [unwired: 3 in, 1 out]
                  }
                }
                n201 = local read "Scans"() -> (w327:i32)
                n202 = Compound Arithmetic op=MULTIPLY(w330, w329, w328, w327) -> (w326:i32)
                n203 = local write "Tab Control"(T3."Image Stack" ("Tab Control")) -> ()
              }
            }
            "TotalSamples" <- w309
            n204 = local read "StackSize"() -> (w314:cluster{"nX":u32, "nY":u32, "nZ":u32})
            n205 = Bundle By Name(cluster=w314, "nX"=w315, "nY"=w303, "nZ"=w316) -> (→"StackSize":cluster{"nX":u32, "nY":u32, "nZ":u32})
          }
          frame #1 {
            n206 = Or(x="SaveStream", y="SaveImage") -> (x .or. y?=w380:bool)
            n207 = case shown="True" w380 {
              tunnel: [w383 w388] -> w379
              frame False {
                (unwired) FALSE
                (unwired) u32 0 ("file handle")
                n208 = local read "StreamInfo"() -> (w385:T5)
                n209 = Bundle By Name(cluster=w385, "Open"=FALSE) -> (w383:T5)
              }
              frame True {
                w389 = "image" ("group name (empty)")
                n210 = local read "Mode"() -> (w391:enum16{"Points", "Volume", "Idle"})
                n211 = local read "NumChans"() -> (w386:u32)
                n212 = local read "Scans"() -> (w387:i32)
                n213 = call <instrlib>:"niHWS Open File.vi"("permissions (0:read only)"=niHWS_Open_File_Permissions_ID."Read/Write/Create New", "file path"="Path") -> ("file handle"=w390:u32)  [unwired: 8 in, 1 out]
                n214 = case shown="\"Volume\"" w391 {
                  tunnel: w390 -> [w413 w429]
                  tunnel: w389 -> [w412 w428]
                  tunnel: w387 -> [_ w414]
                  frame "Points", Default {
                    n215 = local read "Points"() -> (w409:i32[][])
                    n216 = Array Size(array=w409) -> (size(s)=w410:i32[])
                    n217 = call <instrlib>:"niHWS New Wfm Reference.vi"("waveform name (empty)"="points", "group name (empty)"=w412, "file handle in"=w413) -> ("waveform reference"=w406:u32)  [unwired: 6 in, 2 out]
                    n218 = Multiply Array Elements(1:w410) -> (0:w408:i32)
                    n219 = Reshape Array(w409, w408) -> (w407:i32[])
                    n220 = call-poly <instrlib>:"niHWS Write.vi"("data"=w407, "waveform reference in"=w406) -> ()  [unwired: 8 in, 2 out]
                  }
                  frame "Volume" {
                    n221 = local read "Scan Settings"() -> (w427:T4)
                    n222 = call <instrlib>:"niHWS New Wfm Reference.vi"("waveform name (empty)"="volume_settings", "group name (empty)"=w428, "file handle in"=w429) -> ("waveform reference"=w417:u32)  [unwired: 6 in, 2 out]
                    n223 = Unbundle By Name(w427) -> ("XStart"=w426:i32, "XEnd"=w425:i32, "XNum"=w424:i32, "YStart"=w423:i32, "YEnd"=w422:i32, "YNum"=w421:i32, "ZStart"=w420:i32, "ZEnd"=w419:i32, "ZNum"=w415:i32)
                    n224 = Build Array(w426, w425, w424, w423, w422, w421, w420, w419, w415, w414) -> (w418:i32[])
                    n225 = call-poly <instrlib>:"niHWS Write.vi"("data"=w418, "waveform reference in"=w417) -> ()  [unwired: 8 in, 2 out]
                  }
                }
                n226 = call <instrlib>:"niHWS New Wfm Reference.vi"("waveform name (empty)"="stream", "group name (empty)"="stream", "file handle in"=w390) -> ("waveform reference"=w398:u32, "file handle out"=w395:u32)  [unwired: 6 in, 1 out]
                n227 = Build Array(w391, w386) -> (w393:u32[])
                n228 = call <instrlib>:"niHWS New Wfm Reference.vi"("waveform name (empty)"="Mode", "group name (empty)"=w389, "file handle in"=w390) -> ("waveform reference"=w392:u32)  [unwired: 6 in, 2 out]
                n229 = call <instrlib>:"niHWS New Wfm Reference.vi"("waveform name (empty)"="image", "group name (empty)"=w389, "file handle in"=w395) -> ("waveform reference"=w399:u32, "file handle out"=w396:u32)  [unwired: 6 in, 1 out]
                n230 = call-poly <instrlib>:"niHWS Write.vi"("data"=w393, "waveform reference in"=w392) -> ()  [unwired: 8 in, 2 out]
                n231 = local read "StreamInfo"() -> (w400:T5)
                n232 = Bundle By Name(cluster=w400, "Open"=TRUE, "file handle out"=w396, "image reference"=w399, "stream reference"=w398) -> (w388:T5)
              }
            }
            "StreamInfo" <- w379
          }
          frame #2 {
            n233 = local read "FPGA VI Execution Mode"() -> (w435:T6)
            n234 = case shown="\"FPGA Target\", Default" w435 {
              tunnel: w434 -> [w452 _]
              tunnel: w433 -> [w441 w516]
              tunnel: w432 -> [w440 w515]
              tunnel: [w439 w515] -> w431
              tunnel: [w438 w516] -> w430
              frame "FPGA Target", Default {
                n235 = flat-sequence {
                  tunnel: w452 -> [w463]
                  tunnel: [w462] -> w461
                  tunnel: w461 -> [w469]
                  tunnel: [w467] -> w444
                  tunnel: [w477] -> w451
                  tunnel: [w480] -> w448
                  tunnel: [w479] -> w446
                  tunnel: w444 -> [w478]
                  tunnel: [w478] -> w443
                  tunnel: [w476] -> w442
                  tunnel: w451 -> [w493]
                  tunnel: [w493] -> w450
                  tunnel: [w492] -> w449
                  tunnel: w448 -> [w491]
                  tunnel: [w491] -> w447
                  tunnel: w446 -> [w490]
                  tunnel: [w490] -> w445
                  tunnel: w443 -> [w489]
                  tunnel: w442 -> [w492]
                  tunnel: w441 -> [w487]
                  tunnel: w440 -> [w486]
                  tunnel: [w485] -> w439
                  tunnel: [w484] -> w438
                  tunnel: [w482] -> w436
                  tunnel: w450 -> [w501]
                  tunnel: [w499] -> w460
                  tunnel: w449 -> [w498]
                  tunnel: [w497] -> w459
                  tunnel: [w496] -> w458
                  tunnel: w447 -> [w496]
                  tunnel: w445 -> [w495]
                  tunnel: [w495] -> w457
                  tunnel: [w494] -> w437
                  tunnel: w436 -> [w494]
                  tunnel: w460 -> [w510]
                  tunnel: w459 -> [w509]
                  tunnel: [w508] -> w456
                  tunnel: [w507] -> w455
                  tunnel: [w505] -> w454
                  tunnel: w458 -> [w505]
                  tunnel: [w504] -> w453
                  tunnel: w457 -> [w504]
                  tunnel: w437 -> [w503]
                  tunnel: w456 -> [w514]
                  tunnel: w455 -> [w513]
                  tunnel: w454 -> [w512]
                  tunnel: w453 -> [w511]
                  frame #0 {
                    n236 = while {
                      tunnel: w463 -> [w466]
                      tunnel: [w464] -> w462
                      stop <- w465 stop-if-true
                      n237 = xnode "Read/Write Control"("FPGA VI Reference In"=w466) -> ("FPGA VI Reference Out"=w464:T10, "Armed"=w465)  [unwired: 1 in, 1 out]
                    }
                  }
                  frame #1 {
                    n238 = xnode "Read/Write Control"("FPGA VI Reference In"=w469, "ExtAcqTrig"=FALSE) -> ("FPGA VI Reference Out"=w467:T10)  [unwired: 1 in, 1 out]
                    n239 = Wait (ms)(milliseconds to wait=u32 50) -> ()  [unwired: 1 out]
                  }
                  frame #2 {
                    w479 = tag "/PXI1Slot5/PXI_Trig0" ("destination terminal")
                    w480 = tag "/PXI1Slot5/PFI0" ("source terminal")
                    n240 = call-poly <vilib>:"DAQmx Create Virtual Channel.vi"("lines"=tag "PXI1Slot5/port0/line0") -> ("task out"=w475:refnum<k21>, "error out"=w474:errorcluster)  [unwired: 13 in]
                    n241 = Wait (ms)(milliseconds to wait=u32 100) -> ()  [unwired: 1 out]
                    n242 = call-poly <vilib>:"DAQmx Write.vi"("task/channels in"=w475, "auto start"=TRUE, "data"=FALSE, "error in"=w474) -> ("task out"=w477:refnum<k21>, "error out"=w476:errorcluster)  [unwired: 9 in, 1 out]
                    n243 = call <vilib>:"DAQmx Connect Terminals.vi"("source terminal"=w480, "destination terminal"=w479) -> ()  [unwired: 13 in, 1 out]
                  }
                  frame #3 {
                    n244 = xnode "Read/Write Control"("FPGA VI Reference In"=w489, "ExtAcqTrig"=TRUE) -> ("FPGA VI Reference Out"=w482:T10)  [unwired: 1 in, 1 out]
                    n245 = call <vilib>:"DAQmx Start Task.vi"("task/channels in"=w487, "error in"=w486) -> ("task out"=w484:refnum<k21>, "error out"=w485:errorcluster)  [unwired: 12 in]
                    n246 = Wait (ms)(milliseconds to wait=u32 100) -> ()  [unwired: 1 out]
                  }
                  frame #4 {
                    n247 = call-poly <vilib>:"DAQmx Write.vi"("task/channels in"=w501, "data"=TRUE, "error in"=w498) -> ("task out"=w499:refnum<k21>, "error out"=w497:errorcluster)  [unwired: 10 in, 1 out]
                  }
                  frame #5 {
                    w502 = FALSE ("ExtAcqTrig")
                    n248 = xnode "Read/Write Control"("FPGA VI Reference In"=w503, "ExtAcqTrig"=w502, "TriggerAcq"=w502, "Volume Scan"=w502) -> ()  [unwired: 1 in, 2 out]
                    n249 = call-poly <vilib>:"DAQmx Write.vi"("task/channels in"=w510, "data"=FALSE, "error in"=w509) -> ("task out"=w508:refnum<k21>, "error out"=w507:errorcluster)  [unwired: 10 in, 1 out]
                  }
                  frame #6 {
                    n250 = call <vilib>:"DAQmx Disconnect Terminals.vi"("source terminal"=w512, "destination terminal"=w511) -> ()  [unwired: 13 in, 1 out]
                    n251 = call <vilib>:"DAQmx Clear Task.vi"("task in"=w514, "error in"=w513) -> ()  [unwired: 13 in, 1 out]
                  }
                }
              }
              frame "Development Computer with Simulated I/O" {
              }
            }
          }
        }
      }
      frame "Acquire" {
        # "Take data and shuffle between various FIFO's and queues\n(producer loop)"
        n252 = local read "TotalSamples"() -> (w553:u32)
        n253 = local read "Downsample"() -> (w549:i32)
        n254 = local read "PMT Read"() -> (w538:i32)
        n255 = local read "ImCh Read"() -> (w536:i32)
        n256 = Subtract(x=w553, y=w536) -> (x-y=w552:u32)
        n257 = Multiply(x="ImReadSize", y=w549) -> (x*y=w528:i32)
        n258 = Multiply(x=w549, y=w553) -> (x*y=w550:u32)
        n259 = To Unsigned Long Integer(number=w538) -> (unsigned 32bit integer=w548:u32)
        n260 = local read "FPGA VI Execution Mode"() -> (w537:T6)
        n261 = Greater Than 0?(x=w552) -> (x > 0?=w540:bool)
        n262 = Not(x="Abort") -> (.not. x?=w539:bool)
        n263 = Subtract(x=w550, y=w548) -> (x-y=w527:u32)
        n264 = And(x=w539, y=w540) -> (x .and. y?=w541:bool)
        n265 = Max & Min(x=w528, y=w527) -> (min(x,y)=w526:u32)  [unwired: 1 out]
        n266 = local read "PMT Read"() -> (w521:i32)
        n267 = xnode "Read/Write Control"("FPGA VI Reference In"=w530, "Abort"="Abort") -> ()  [unwired: 1 in, 2 out]
        n268 = Select(t=u32 0, s="Abort", f=w526) -> (s? t:f=w542:u32)
        n269 = Equal To 0?(x=w521) -> (x = 0?=w520:bool)
        n270 = local read "NumChans"() -> (w522:u32)
        n271 = Select(t=w519, s=w520, f=0.0) -> (s? t:f=w517:dbl)
        n272 = case shown="True" w541 {
          tunnel: w530 -> [_ w636]
          tunnel: w536 -> [_ _]
          tunnel: "ImReadSize" -> [_ w637]
          tunnel: [TRUE FALSE] -> w534
          tunnel: w552 -> [_ w638]
          tunnel: w536 -> [_ w625]
          frame False {
          }
          frame True {
            n273 = local read "NumChans"() -> (w631:u32)
            n274 = Max & Min(x=w637, y=w638) -> (min(x,y)=w635:u32)  [unwired: 1 out]
            n275 = Multiply(x=w631, y=w635) -> (x*y=w634:u32)
            n276 = xnode "Invoke Method"("FPGA VI Reference In"=w636, "Number of Elements"=w634, "Timeout (ms)"=5) -> ("error out"=w628:errorcluster, "Data"=w623:void[], "Elements Remaining"=→"ImCh Backlog")  [unwired: 1 in, 1 out]
            n277 = Array Size(array=w623) -> (size(s)=w632:i32)
            n278 = call <vilib>:"Clear Errors.vi"("error in (no error)"=w628) -> ()  [unwired: 6 in, 1 out]
            n279 = local read "voxel queue"() -> (w624:refnum<queue>)
            n280 = Divide(x=w632, y=w631) -> (x/y=w629:dbl)
            n281 = To Unsigned Long Integer(number=w629) -> (unsigned 32bit integer=w630:u32)
            n282 = Add(x=w630, y=w625) -> (x+y=→"ImCh Read":u32)
            n283 = Enqueue Element(queue=w624, element=w623) -> ()  [unwired: 2 in, 3 out]
          }
        }
        n284 = Multiply(x=w522, y=w517) -> (x*y=w525:dbl)
        n285 = Divide(x=w525, y=2 ("x")) -> (x/y=w524:dbl)
        n286 = case shown="1, Default" w542 {
          selector: w542 -> [_ w590]
          tunnel: [w560 w602] -> w558
          tunnel: w545 -> [w561 w599]
          tunnel: w544 -> [w563 w601]
          tunnel: [w562 w600] -> w546
          tunnel: w530 -> [_ w596]
          tunnel: w537 -> [_ w593]
          tunnel: [TRUE FALSE] -> w531
          tunnel: w517 -> [_ w588]
          tunnel: w524 -> [_ w586]
          frame 0 {
            n287 = local read "FPGA VI Execution Mode"() -> (w564:T6)
            n288 = case shown="\"FPGA Target\", Default" w564 {
              tunnel: w563 -> [w570 w579]
              tunnel: [w566 w579] -> w562
              tunnel: [w565 w578] -> w560
              tunnel: w561 -> [w571 w578]
              frame "FPGA Target", Default {
                n289 = property class="DAQmx Task"(reference=w571, error in=w570) -> (reference out=w568:refnum<k21>, error out=w567:errorcluster, "Done"=w569:bool)
                n290 = case shown="True" w569 {
                  tunnel: w568 -> [w575 w576]
                  tunnel: w567 -> [w574 w577]
                  tunnel: [w573 w577] -> w566
                  tunnel: [w572 w576] -> w565
                  frame False {
                    n291 = call <vilib>:"DAQmx Stop Task.vi"("task/channels in"=w575, "error in"=w574) -> ("task out"=w572:refnum<k21>, "error out"=w573:errorcluster)  [unwired: 12 in]
                  }
                  frame True {
                  }
                }
              }
              frame "Development Computer with Simulated I/O" {
              }
            }
          }
          frame 1, Default {
            n292 = Add(x=w588, y=w590) -> (x+y=w589:dbl)
            n293 = case shown="\"FPGA Target\", Default" w593 {
              tunnel: [w612 w621] -> w602
              tunnel: w601 -> [w611 w620]
              tunnel: [w609 w618] -> w587
              tunnel: w589 -> [w608 w617]
              tunnel: [w607 w620] -> w600
              tunnel: w599 -> [w605 w621]
              frame "FPGA Target", Default {
                n294 = property class="DAQmx Read"(reference=w605) -> ("AvailSampPerChan"=→"PMT Backlog":u32)  [unwired: 1 in, 2 out]
                n295 = call-poly <vilib>:"DAQmx Read.vi"("task/channels in"=w605, "number of samples per channel"=w608, "timeout"=2.0, "error in"=w611) -> ("task out"=w612:refnum<k21>, "data"=w609:i32[], "error out"=w607:errorcluster)  [unwired: 9 in]
              }
              frame "Development Computer with Simulated I/O" {
                n296 = local read "NumChans"() -> (w614:u32)
                n297 = Divide(x=w617, y=u32 2) -> (x/y=w615:dbl)
                n298 = Divide(x=w615, y=w614) -> (x/y=w613:dbl)
                n299 = call-poly <vilib>:"Ramp Pattern.vi"("samples"=w613) -> ("Ramp Pattern"=w619:dbl[])  [unwired: 9 in, 1 out]
                n300 = To Unsigned Long Integer(number=w619) -> (unsigned 32bit integer=w618:u32[])
              }
            }
            n301 = Split 1D Array(array=w587, index=w586) -> (second subarray=w585:u32[])  [unwired: 1 out]
            n302 = local read "NumChans"() -> (w584:u32)
            n303 = xnode "Invoke Method"("FPGA VI Reference In"=w596, "Data"=w585, "Timeout (ms)"=-1) -> ("Empty Elements Remaining"=→"PMT FIFO Space")  [unwired: 1 in, 2 out]
            n304 = Array Size(array=w585) -> (size(s)=w595:i32)
            n305 = Multiply(x=w595, y=2) -> (x*y=w583:i32)
            n306 = Divide(x=w583, y=w584) -> (x/y=w582:dbl)
            n307 = local read "SaveStream"() -> (w592:bool)
            n308 = local read "PMT Read"() -> (w580:i32)
            n309 = Add(x=w580, y=w582) -> (x+y=→"PMT Read":dbl)
            n310 = case shown="True" w592 {
              tunnel: w585 -> [_ w604]
              frame False {
              }
              frame True {
                n311 = local read "raw out"() -> (w603:refnum<queue>)
                n312 = Enqueue Element(queue=w603, element=w604) -> ()  [unwired: 2 in, 3 out]
              }
            }
          }
        }
        n313 = local read "Abort"() -> (w533:bool)
        n314 = And(x=w531, y=w534) -> (x .and. y?=w532:bool)
        n315 = Unbundle By Name(w546) -> ("status"=w547:bool)
        n316 = Compound Arithmetic op=OR(w547, w532, w533) -> (w551:bool)
        n317 = Select(t=T2."End Acquire", s=w551, f=T2."Acquire") -> (s? t:f=w557:T2)
        "Throwaway Samples" <- w519
      }
      frame "End Acquire" {
        w655 = T14 2 items=["no dialog", "OK message", "continue or stop message", "OK message + warnings", "continue/stop + warnings"] ("type of dialog (OK msg:1)")
        n318 = local read "Processing"() -> (w643:bool)
        n319 = xnode "Read/Write Control"("FPGA VI Reference In"=w653, "TriggerAcq"=FALSE) -> ()  [unwired: 1 in, 2 out]
        n320 = Not(x=w643) -> (.not. x?=w644:bool)
        n321 = call <vilib>:"General Error Handler.vi"("type of dialog (OK msg:1)"=w655, "error in (no error)"=w656) -> ("error out"=w651:errorcluster)  [unwired: 9 in, 4 out]
        n322 = feedback-in #5(w644) -> ()
        n323 = feedback #5() -> (w645:bool)  [unwired: 1 in]
        n324 = feedback-in #6(w645) -> ()
        n325 = feedback #6() -> (w646:bool)  [unwired: 1 in]
        n326 = Not(x=w643) -> (.not. x?=w648:bool)
        n327 = feedback-in #7(w643) -> ()
        n328 = feedback #7() -> (w647:bool)  [unwired: 1 in]
        n329 = Compound Arithmetic op=AND(w644, w645, w646) -> (w641:bool)
        n330 = And(x=w648, y=w647) -> (x .and. y?=w642:bool)
        n331 = Or(x=w642, y=w641) -> (x .or. y?=w640:bool)
        n332 = case shown="True" w640 {
          tunnel: [T2."Reset" T2."End Acquire"] -> w649
          frame True {
            n333 = local read "StreamInfo"() -> (w659:T5)
            n334 = Bundle By Name(cluster=w659, "Open"=FALSE) -> (w661:T5)
            n335 = Unbundle By Name(w659) -> ("file handle out"=w662:u32, "Open"=w657:bool)
            n336 = local write "StreamInfo"(w661) -> ()
            n337 = case shown="True" w657 {
              tunnel: w662 -> [_ w663]
              frame False {
              }
              frame True {
                n338 = call <instrlib>:"niHWS Close File.vi"("file handle"=w663) -> ()  [unwired: 10 in, 1 out]
              }
            }
          }
          frame False {
            n339 = Wait (ms)(milliseconds to wait=u32 50) -> ()  [unwired: 1 out]
          }
        }
      }
    }
    "Loop Count" <- w148
    "Host State" <- w143
  }
  n340 = while {
    shift-right: [w668] -> _
    shift-left: _ -> [w667]
    shift-right: [w670] -> _
    shift-left: _ -> [w671]
    stop <- w666 stop-if-true
    n341 = event shown="[1] \"Section\": Value Change" {
      selector: _ -> [_ _ _ _ _]
      dyn-events: _ -> [_ _ _ _ _]
      timeout: 500 -> [_ _ _ _ _]
      tunnel: w671 -> [w684 w700 w718 w760 w768]
      tunnel: [w685 w700 w711 w759 w767] -> w670
      tunnel: [w675 w698 w712 w758 w772] -> w668
      tunnel: w667 -> [w675 w698 w712 w758 w770]
      event Timeout {
        n342 = event-data() -> ()  [unwired: 1 in, 2 out]
        n343 = local read "Host State"() -> (w682:T2)
        n344 = local read "Mode"() -> (w680:enum16{"Points", "Volume", "Idle"})
        n345 = property on="ImCh1 2" class="ImageControl"() -> ("ROI"=w683:T15)  [unwired: 2 in, 2 out]
        n346 = Equal?(x=enum16{"Points", "Volume", "Idle"}."Volume", y=w680) -> (x = y?=w678:bool)
        n347 = Not Equal?(x=w682, y=T2."Idle") -> (x != y?=w677:bool)
        n348 = Replace Array Subset(array=w684, new element=w683) -> (w685:T16)  [unwired: 1 in]
        n349 = And(x=w677, y=w678) -> (x .and. y?=w676:bool)
        n350 = Divide(x="Max", y=255.0) -> (x/y=w672:dbl)
        n351 = case shown="True" w676 {
          tunnel: w675 -> [_ w688]
          tunnel: w672 -> [_ w686]
          frame False {
          }
          frame True {
            n352 = local read "ImData"() -> (w687:i32[][])
            n353 = local read "ImCh1 2"() -> (w693:T9)
            n354 = local read "ImCh2 2"() -> (w692:T9)
            n355 = Divide(x=w687, y=w686) -> ()  [unwired: 1 out]
            n356 = call "UpdateStack.vi"("Scan Settings"=w688, "Section"="Section", "ImData"=w687, "Im2 2"=w692, "Im1 In"=w693) -> ("Im2 Out"=→"ImCh2 2":T9, "Im1 Out"=→"ImCh1 2":T9)  [unwired: 5 in]
          }
        }
      }
      event "Section": Value Change {
        n357 = event-data() -> ("NewVal"=w699:i32)  [unwired: 1 in, 4 out]
        n358 = local read "Max"() -> (w695:u32)
        n359 = Divide(x=w695, y=u8 255) -> (x/y=w696:dbl)
        n360 = local read "Display Data"() -> (w697:bool)
        n361 = case shown="True" w697 {
          tunnel: w699 -> [_ w706]
          tunnel: w698 -> [_ w705]
          tunnel: w696 -> [_ w702]
          frame False {
          }
          frame True {
            n362 = local read "ImData"() -> (w704:i32[][])
            n363 = local read "ImCh1 2"() -> (w709:T9)
            n364 = local read "ImCh2 2"() -> (w710:T9)
            n365 = Divide(x=w704, y=w702) -> (x/y=w703:dbl[][])
            n366 = call "UpdateStack.vi"("Scan Settings"=w705, "Section"=w706, "ImData"=w703, "Im2 2"=w710, "Im1 In"=w709) -> ("Im2 Out"=w708:T9, "Im1 Out"=w707:T9)  [unwired: 5 in]
            n367 = local write "ImCh2 2"(w708) -> ()
            n368 = local write "ImCh1 2"(w707) -> ()
          }
        }
        n369 = Index Array(array=w700, index=w699) -> (element=w701:T15)
        n370 = property on="ImCh1 2" class="ImageControl"("ROI"=w701) -> ()  [unwired: 2 in, 2 out]
      }
      event "ImCh1 2": Mouse Down; "ImCh2 2": Mouse Up {
        n371 = event-data() -> ()  [unwired: 1 in, 7 out]
        n372 = local read "Section"() -> (w716:i32)
        n373 = property on="ImCh1 2" class="ImageControl"() -> ("ROI"=w717:T15)  [unwired: 2 in, 2 out]
        n374 = Replace Array Subset(array=w718, new element=w717, index=w716) -> (w711:T16)
        n375 = for {
          tunnel: w711 -> [w725] mode=indexing
          shift-right: [w721] -> w715
          shift-left: i32[][] [] -> [w722]
          tunnel: w712 -> [w720]
          tunnel: "GridPoints" -> [w719]
          i -> [w723]
          n376 = Unbundle By Name(w725) -> ("Contours"=w724:T17)
          n377 = for {
            tunnel: w724 -> [w733] mode=indexing
            tunnel: w723 -> [w729]
            shift-right: [w728] -> w721
            shift-left: w722 -> [w730]
            tunnel: w720 -> [w727]
            tunnel: w719 -> [w726]
            n378 = Unbundle By Name(w733) -> ("ROI Type"=w732:u32, "Points"=w731:i32[])
            n379 = case shown="1" w732 {
              tunnel: w731 -> [_ w741 w749 w754]
              tunnel: w730 -> [w734 w739 w745 w757]
              tunnel: w729 -> [_ w740 w748 w756]
              tunnel: [w734 w738 w743 w755] -> w728
              tunnel: w727 -> [_ w736 w747 w753]
              tunnel: w726 -> [_ _ w742 w750]
              frame 0, Default {
              }
              frame 1 {
                n380 = Build Array (concatenate)(w741, w740) -> (w735:i32[])
                n381 = call "PointToSetting.vi"("Clicked"=w735, "Scan Settings"=w736) -> ("Setting"=w737:i32[])  [unwired: 9 in]
                n382 = Build Array (concatenate)(w739, w737) -> (w738:i32[][])
              }
              frame 2 {
                n383 = Build Array (concatenate)(w749, w748) -> (w746:i32[])
                n384 = call "LineToSetting.vi"("GridSize"=w742, "Line"=w746, "Scan Settings"=w747) -> ("Settings"=w744:i32[][])  [unwired: 8 in]
                n385 = Build Array (concatenate)(w745, w744) -> (w743:i32[][])
              }
              frame 3 {
                n386 = Build Array (concatenate)(w754, w756) -> (w751:i32[])
                n387 = call "BoxToSetting.vi"("GridSize"=w750, "Line"=w751, "Scan Settings"=w753) -> ("Settings"=w752:i32[][])  [unwired: 8 in]
                n388 = Build Array (concatenate)(w757, w752) -> (w755:i32[][])
              }
            }
          }
        }
        n389 = local write "Points"(w715) -> ()
      }
      event "ClearPoints": Value Change {
        n390 = event-data() -> ("NewVal"=w761:bool)  [unwired: 1 in, 4 out]
        n391 = case shown="True" w761 {
          tunnel: w760 -> [w762 _]
          tunnel: [w762 w766] -> w759
          tunnel: w758 -> [_ w764]
          frame False {
          }
          frame True {
            w765 = T15 {"Global Rectangle"=[], "Contours"=[]} ("ROI")
            n392 = Unbundle By Name(w764) -> ("ZNum"=w763:i32)
            n393 = Initialize Array(w765, w763) -> (w766:T16)
            n394 = property on="ImCh1 2" class="ImageControl"("ROI"=w765) -> ()  [unwired: 2 in, 2 out]
          }
        }
      }
      event "Volume Scan": Value Change {
        n395 = event-data() -> ()  [unwired: 1 in, 5 out]
        n396 = local read "Scan Settings"() -> (w771:T4)
        n397 = Equal?(x=w771, y=w770) -> (x = y?=w769:bool)
        n398 = case shown="False" w769 {
          tunnel: w771 -> [w775 w778]
          tunnel: [w775 w778] -> w772
          tunnel: [w774 w777] -> w767
          tunnel: w768 -> [_ w777]
          frame False {
            w776 = T15 {"Global Rectangle"=[], "Contours"=[]} ("ROI")
            n399 = Unbundle By Name(w775) -> ("ZNum"=w773:i32)  [unwired: 2 out]
            n400 = property on="Section" class="Scroll (strict)"("DocMax"=w773) -> ()  [unwired: 2 in, 2 out]
            n401 = Initialize Array(w776, w773) -> (w774:T16)
            n402 = property on="ImCh1 2" class="ImageControl"("ROI"=w776) -> ()  [unwired: 2 in, 2 out]
          }
          frame True {
          }
        }
      }
    }
    n403 = local read "Stop"() -> (w666:bool)
  }
  n404 = case shown="\"FPGA Target\", Default" w19 {
    tunnel: [w779 w782] -> w32
    tunnel: w30 -> [w780 w782]
    frame "FPGA Target", Default {
      w781 = T11 5 items=["PXI_Trig0", "PXI_Trig1", "PXI_Trig2", "PXI_Trig3", "PXI_Trig4", "PXI_Trig5", "PXI_Trig6", "PXI_Trig7"] ("Trigger")
      n405 = xnode "Invoke Method"("FPGA VI Reference In"=w780, "Trigger"=w781) -> ("FPGA VI Reference Out"=w779:T10)  [unwired: 1 in, 1 out]
    }
    frame "Development Computer with Simulated I/O" {
    }
  }
  n406 = call <vilib>:"DAQmx Stop Task.vi"("task/channels in"=w28, "error in"=w27) -> ()  [unwired: 12 in, 2 out]
  n407 = xnode "Close FPGA VI Reference"("FPGA VI Reference In"=w32) -> ()  [unwired: 1 in, 1 out]
